vi "I_Method_Current_Transaction.vi"(8 "error in (no error)":errorcluster, 11 "Interface Current Transaction in":refnum<class "Interface Display_Console_Actor.lvclass">) -> (0 "error out":errorcluster, 3 "Interface Current Transaction out":refnum<class "Interface Display_Console_Actor.lvclass">)   [LabVIEW 2025]
uses:
  Interface Display_Console_Actor.lvclass
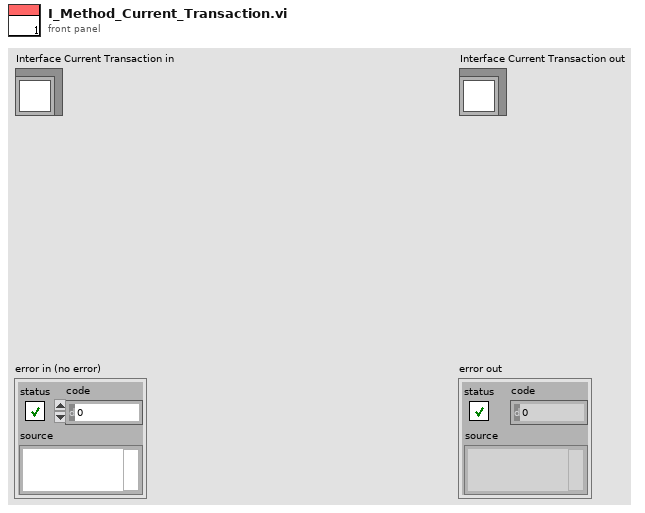
[diagram p1: front panel]
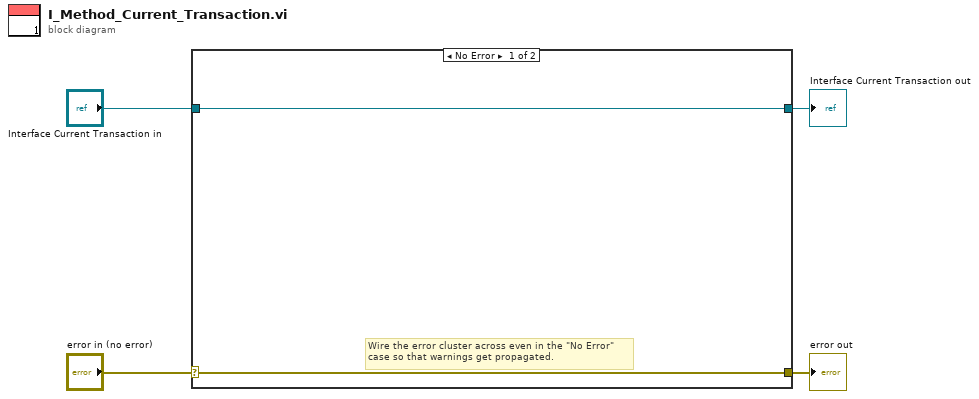
[diagram p0: block diagram]
diagram:
  n1 = case shown="No Error" "error in (no error)" {
    selector: "error in (no error)" -> [w5 w8]
    tunnel: [w5 w8] -> w3
    tunnel: [w6 w7] -> w1
    tunnel: "Interface Current Transaction in" -> [w6 w7]
    frame No Error {
      # "Wire the error cluster across even in the \"No Error\"\ncase so that warnings get propagated."
    }
    frame Error {
    }
  }
  "error out" <- w3
  "Interface Current Transaction out" <- w1
